vi "evo irimager set radiation parameters.vi"(9 "tAmbient":sgl, 10 "transmissivity":sgl, 11 "emissivity":sgl) -> (3 "function return":i32)   [LabVIEW 2012, in "libirimager_direct_binding.lvlib"]
doc: "__IRDIRECTSDK_API__ int evo_irimager_set_radiation_parameters(float emissivity, float transmissivity, float tAmbient=-999.f);"
uses:
  libirimager_direct_binding.lvlib
  Users/HelmutEngelhardt/Documents/labview_2017/labview/libirimager.dll
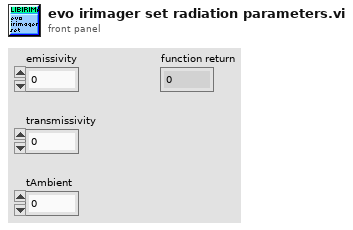
[diagram p1: front panel]
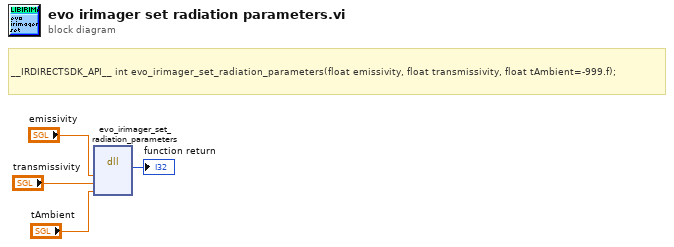
[diagram p0: block diagram]
diagram:
  # "__IRDIRECTSDK_API__ int evo_irimager_set_radiation_parameters(float emissivity, float transmissivity, float tAmbient=-999.f);"
  n1 = dll-call lib="C:/Users/HelmutEngelhardt/Documents/labview_2017/labview/libirimager.dll" fn="evo_irimager_set_radiation_parameters"("emissivity"="emissivity", "transmissivity"="transmissivity", "tAmbient"="tAmbient") -> ("Rückgabetyp"=→"function return":i32)  [unwired: 6 in, 2 out]
